vi "DAQ Engine.vi"(11 "Sequence Context In":refnum<k7>) -> (0 "error out":errorcluster)   [LabVIEW 2023, in "LTT_TeststandSteptypes.lvlib"]
doc: "This VI is DAQ Engine Thread Driver"
uses:
  LTT_TeststandSteptypes.lvlib
  HardwareAbstractionLayer_LVOOP/Database/Database.lvclass
  HardwareAbstractionLayer_LVOOP/Database/SQL Public VI/Control/DB Options.ctl
  HardwareAbstractionLayer_LVOOP/Teststand/Teststand.lvclass
  <vilib>/addons/TestStand/_TSUtility.llb/TestStand - Set Property Value (String).vi
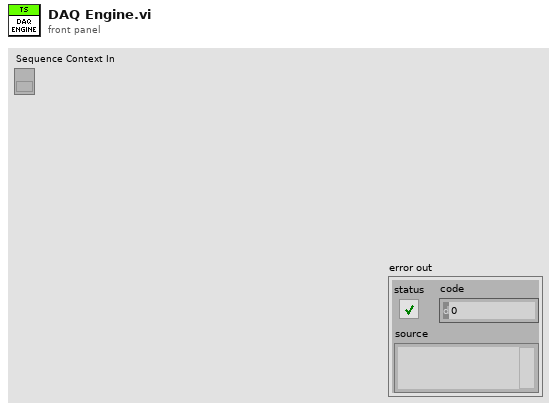
[diagram p1: front panel]
types:
  T1 = typedef "HardwareAbstractionLayer_LVOOP.lvlib/Database.lvclass/DB Options.ctl" = enum16{"Init", "Select Data", "Insert Data", "Update Data", "Delete Data", "Execute Query", "Create Schema", "Create Table", "List Tables", "List Columns", "Close"}
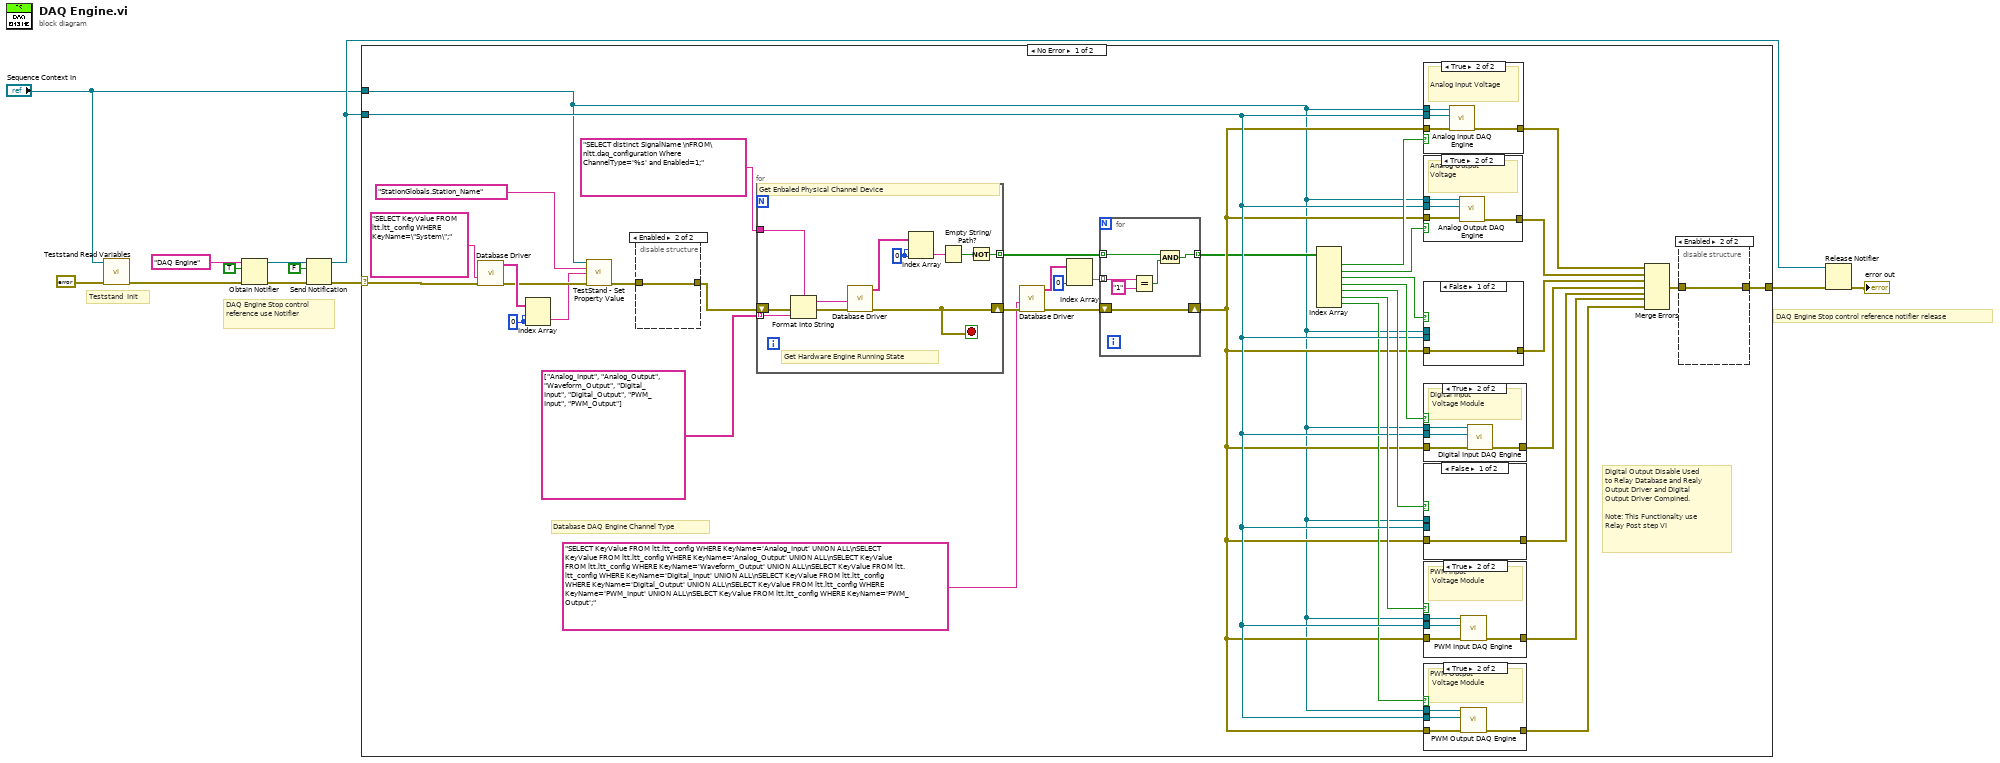
[diagram p0: block diagram]
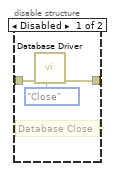
[diagram p2: hidden frame]
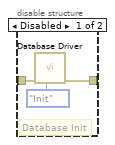
[diagram p3: hidden frame]
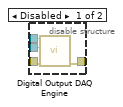
[diagram p9: hidden frame]
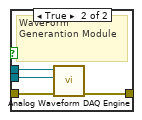
[diagram p11: hidden frame]
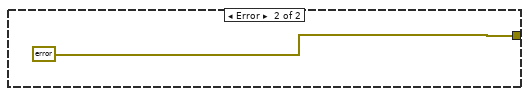
[diagram p12: hidden frame]
diagram:
  # "Teststand  Init"
  # "DAQ Engine Stop control reference notifier release"
  # "DAQ Engine Stop control reference use Notifier"
  n1 = call "Teststand Read Variables.vi"("error in"=errorcluster {"status"=FALSE, "code"=0, "source"=""}, "Sequence Context In"="Sequence Context In") -> ("error out"=w2:errorcluster)  [unwired: 9 in]
  n2 = Obtain Notifier(name (unnamed)="DAQ Engine", notification data type=TRUE, error in (no error)=w2) -> (notifier out=w8:refnum<notifier>, error out=w7:errorcluster)  [unwired: 1 in, 1 out]
  n3 = Send Notification(notification=FALSE, notifier=w8, error in (no error)=w7) -> (notifier out=w5:refnum<notifier>, error out=w4:errorcluster)
  n4 = case shown="No Error" w4 {
    selector: w4 -> [w21 _]
    tunnel: [w46 errorcluster {"status"=TRUE, "code"=0, "source"="Database Error. Please check the database connection"} ("error IO")] -> w10
    tunnel: w5 -> [w34 _]
    tunnel: "Sequence Context In" -> [w17 _]
    frame No Error {
      w18 = 0 ("disabled index (col)")
      # "Digital Output Disable Used\nto Relay Database and Realy Output Driver and Digital Output Driver Compined.\n\nNote: This Functionalty use Relay Post step VI"
      # "Database DAQ Engine Channel Type"
      n5 = call "Database Driver.vi"("error in"=w21, "SQL query"="SELECT KeyValue FROM ltt.ltt_config WHERE KeyName=\"System\";") -> ("error out"=w16:errorcluster, "data"=w19:string[][])  [unwired: 6 in, 2 out]
      n6 = Index Array(array=w19, index (row)=w18, index (col)=w18) -> (element=w14:string)
      n7 = call-poly <vilib>:"TestStand - Set Property Value.vi"("Sequence Context In"=w17, "Lookup String"="StationGlobals.Station_Name", "New Value"=w14, "error in (no error)"=w16) -> ("error out"=w15:errorcluster)  [unwired: 10 in, 1 out]
      n8 = disable-structure shown="Enabled" {
        disable-tunnel: [w57 w58] -> w48
        disable-tunnel: w15 -> [w55 w58]
        frame Disabled {
          # "Database Init"
          n9 = call "Database Driver.vi"("Options"=DB_Options."Init", "error in"=w55) -> ("error out"=w57:errorcluster)  [unwired: 6 in, 3 out]
        }
        frame Enabled {
        }
      }
      n10 = for {
        tunnel: "SELECT distinct SignalName \nFROM\nltt.daq_configuration Where ChannelType='%s' and Enabled=1;" -> [w85]
        tunnel: string[] ["Analog_Input", "Analog_Output", "Waveform_Output", "Digital_Input", "Digital_Output", "PWM_Input", "PWM_Output"] -> [w84] mode=indexing
        tunnel: [w77] -> w23 mode=indexing
        shift-right: [w78] -> w30
        shift-left: w48 -> [w76]
        stop <- w78 stop-if-true
        w83 = 0 ("disabled index (col)")
        # "Get Hardware Engine Running State"
        # "Get Enbaled Physical Channel Device"
        n11 = Format Into String(format string=w85, error in=w76, w84) -> (resulting string=w80:string, error out=w75:errorcluster)  [unwired: 1 in]
        n12 = call "Database Driver.vi"("error in"=w75, "SQL query"=w80) -> ("error out"=w78:errorcluster, "data"=w79:string[][])  [unwired: 6 in, 2 out]
        n13 = Index Array(array=w79, index (row)=w83, index (col)=w83) -> (element=w82:string)
        n14 = Empty String/Path?(string/path=w82) -> (empty?=w81:bool)
        n15 = Not(x=w81) -> (.not. x?=w77:bool)
      }
      n16 = call "Database Driver.vi"("error in"=w30, "SQL query"="SELECT KeyValue FROM ltt.ltt_config WHERE KeyName='Analog_Input' UNION ALL\nSELECT KeyValue FROM ltt.ltt_config WHERE KeyName='Analog_Output' UNION ALL\nSELECT KeyValue FROM ltt.ltt_config WHERE KeyName='Waveform_Output' UNION ALL\nSELECT KeyValue FROM ltt.ltt_config WHERE KeyName='Digital_Input' UNION ALL\nSELECT KeyValue FROM ltt.ltt_config WHERE KeyName='Digital_Output' UNION ALL\nSELECT KeyValue FROM ltt.ltt_config WHERE KeyName='PWM_Input' UNION ALL\nSELECT KeyValue FROM ltt.ltt_config WHERE KeyName='PWM_Output';") -> ("error out"=w25:errorcluster, "data"=w28:string[][])  [unwired: 6 in, 2 out]
      n17 = Index Array(array=w28, index (col)=0 ("disabled index (col)")) -> (element=w26:string[])  [unwired: 1 in]
      n18 = for {
        tunnel: w26 -> [w63] mode=indexing
        shift-right: [w64] -> w24
        shift-left: w25 -> [w64]
        tunnel: w23 -> [w60] mode=indexing
        tunnel: [w59] -> w22 mode=indexing
        n19 = Equal?(x=w63, y="1") -> (x = y?=w61:bool)
        n20 = And(x=w60, y=w61) -> (x .and. y?=w59:bool)
      }
      n21 = Index Array(array=w22) -> (element #1=w45:bool, element #2=w44:bool, element #3=w43:bool, element #4=w39:bool, element #5=w37:bool, element #6=w35:bool, element #7=w33:bool)  [unwired: 7 in]
      n22 = case shown="True" w45 {
        tunnel: w24 -> [w70 w74]
        tunnel: [w70 w73] -> w42
        tunnel: w34 -> [_ w72]
        tunnel: w17 -> [_ w71]
        frame False {
        }
        frame True {
          # "Analog Input Voltage"
          n23 = call "Analog Input DAQ Engine.vi"("error in"=w74, "DAQ Engine"=w72, "Sequence Context In"=w71) -> ("error out"=w73:errorcluster)  [unwired: 8 in]
        }
      }
      n24 = case shown="True" w44 {
        tunnel: w24 -> [w65 w69]
        tunnel: [w65 w68] -> w41
        tunnel: w34 -> [_ w67]
        tunnel: w17 -> [_ w66]
        frame False {
        }
        frame True {
          # "Analog Output Voltage"
          n25 = call "Analog Output DAQ Engine.vi"("error in"=w69, "DAQ Engine"=w67, "Sequence Context In"=w66) -> ("error out"=w68:errorcluster)  [unwired: 8 in]
        }
      }
      n26 = case shown="False" w43 {
        tunnel: w24 -> [w111 w115]
        tunnel: [w111 w114] -> w40
        tunnel: w34 -> [_ w113]
        tunnel: w17 -> [_ w112]
        frame False {
        }
        frame True {
          # "WaveForm Generantion Module"
          n27 = call "Analog Waveform DAQ Engine.vi"("error in"=w115, "DAQ Engine"=w113, "Sequence Context In"=w112) -> ("error out"=w114:errorcluster)  [unwired: 8 in]
        }
      }
      n28 = case shown="True" w39 {
        tunnel: w34 -> [_ w108]
        tunnel: w24 -> [w106 w110]
        tunnel: [w106 w109] -> w38
        tunnel: w17 -> [_ w107]
        frame False {
          # "Digital Input\n Voltage Module"
        }
        frame True {
          # "Digital Input\n Voltage Module"
          n29 = call "Digital Input DAQ Engine.vi"("error in"=w110, "DAQ Engine"=w108, "Sequence Context In"=w107) -> ("error out"=w109:errorcluster)  [unwired: 8 in]
        }
      }
      n30 = case shown="False" w37 {
        tunnel: w34 -> [_ w100]
        tunnel: w24 -> [w96 w99]
        tunnel: [w96 w98] -> w36
        tunnel: w17 -> [_ w97]
        frame False {
        }
        frame True {
          # "Digital Output\n Voltage Module"
          n31 = disable-structure shown="Enabled" {
            disable-tunnel: w100 -> [w104 _]
            disable-tunnel: w99 -> [w103 w105]
            disable-tunnel: [w102 w105] -> w98
            disable-tunnel: w97 -> [w101 _]
            frame Disabled {
              n32 = call "Digital Output DAQ Engine.vi"("error in"=w103, "DAQ Engine"=w104, "Sequence Context In"=w101) -> ("error out"=w102:errorcluster)  [unwired: 8 in]
            }
            frame Enabled {
            }
          }
        }
      }
      n33 = case shown="True" w35 {
        tunnel: w34 -> [_ w95]
        tunnel: w24 -> [w91 w94]
        tunnel: [w91 w93] -> w32
        tunnel: w17 -> [_ w92]
        frame False {
        }
        frame True {
          # "PWM Input\n Voltage Module"
          n34 = call "PWM Input DAQ Engine.vi"("error in"=w94, "DAQ Engine"=w95, "Sequence Context In"=w92) -> ("error out"=w93:errorcluster)  [unwired: 8 in]
        }
      }
      n35 = case shown="True" w33 {
        tunnel: w34 -> [_ w90]
        tunnel: w24 -> [w86 w89]
        tunnel: [w86 w88] -> w31
        tunnel: w17 -> [_ w87]
        frame False {
        }
        frame True {
          # "PWM Output\n Voltage Module"
          n36 = call "PWM Output DAQ Engine.vi"("error in"=w89, "DAQ Engine"=w90, "Sequence Context In"=w87) -> ("error out"=w88:errorcluster)  [unwired: 8 in]
        }
      }
      n37 = Merge Errors(w42, w41, w40, w38, w36, w32, w31) -> (w47:errorcluster)
      n38 = disable-structure shown="Enabled" {
        disable-tunnel: w47 -> [w53 w54]
        disable-tunnel: [w51 w54] -> w46
        frame Disabled {
          # "Database Close"
          n39 = call "Database Driver.vi"("Options"=DB_Options."Close", "error in"=w53) -> ("error out"=w51:errorcluster)  [unwired: 6 in, 3 out]
        }
        frame Enabled {
        }
      }
    }
    frame Error {
    }
  }
  n40 = Release Notifier(notifier=w5, error in (no error)=w10) -> (error out=→"error out":errorcluster)  [unwired: 1 in, 2 out]
